vi "InitAngle.vi"(8 "error in (no error)":errorcluster) -> (0 "error out":errorcluster, 3 "AngleTable":dbl[](array[numeric]))   [LabVIEW 2019]
uses:
  <vilib>/Utility/config.llb/Read Key (Double).vi
  <vilib>/Utility/config.llb/NI_LVConfig.lvlib
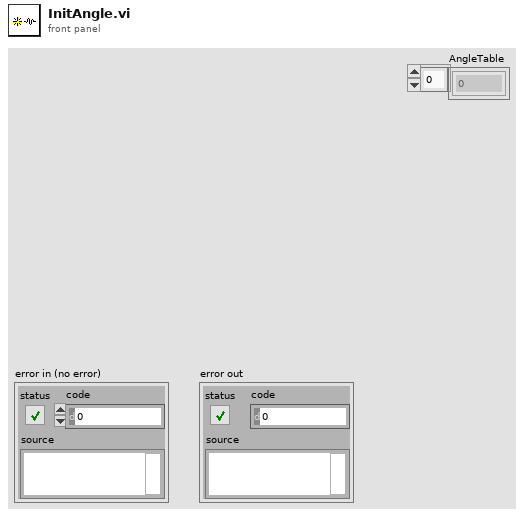
[diagram p1: front panel]
types:
  T1 = typedef "NI_LVConfig.lvlib/Config Data RefNum.ctl" = refnum<k1>
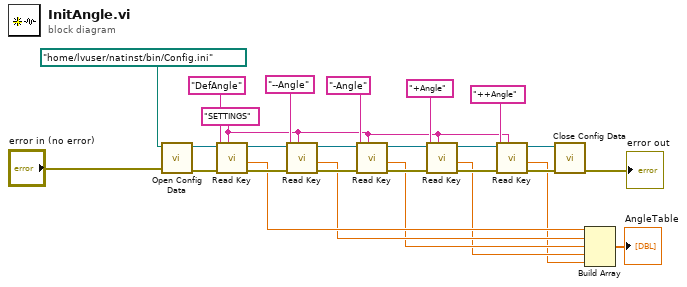
[diagram p0: block diagram]
diagram:
  w19 = "SETTINGS" ("section")
  n1 = call <vilib>:"Open Config Data.vi"("error in (no error)"="error in (no error)", "configuration file path"=path "/home/lvuser/natinst/bin/Config.ini") -> ("error out"=w13:errorcluster, "refnum"=w7:T1)  [unwired: 7 in, 1 out]
  n2 = call-poly <vilib>:"Read Key.vi"("section"=w19, "error in (no error)"=w13, "key"="DefAngle", "refnum"=w7) -> ("error out"=w14:errorcluster, "value"=w6:dbl, "refnum out"=w8:T1)  [unwired: 4 in, 1 out]
  n3 = call-poly <vilib>:"Read Key.vi"("section"=w19, "error in (no error)"=w14, "key"="--Angle", "refnum"=w8) -> ("error out"=w15:errorcluster, "value"=w5:dbl, "refnum out"=w9:T1)  [unwired: 4 in, 1 out]
  n4 = call-poly <vilib>:"Read Key.vi"("section"=w19, "error in (no error)"=w15, "key"="-Angle", "refnum"=w9) -> ("error out"=w16:errorcluster, "value"=w4:dbl, "refnum out"=w10:T1)  [unwired: 4 in, 1 out]
  n5 = call-poly <vilib>:"Read Key.vi"("section"=w19, "error in (no error)"=w16, "key"="+Angle", "refnum"=w10) -> ("error out"=w17:errorcluster, "value"=w3:dbl, "refnum out"=w11:T1)  [unwired: 4 in, 1 out]
  n6 = call-poly <vilib>:"Read Key.vi"("section"=w19, "error in (no error)"=w17, "key"="++Angle", "refnum"=w11) -> ("error out"=w18:errorcluster, "value"=w2:dbl, "refnum out"=w12:T1)  [unwired: 4 in, 1 out]
  n7 = call <vilib>:"Close Config Data.vi"("error in (no error)"=w18, "refnum"=w12) -> ("error out"=→"error out":errorcluster)  [unwired: 8 in, 1 out]
  n8 = Build Array(w6, w5, w4, w3, w2) -> (→"AngleTable":dbl[])
